vi "GetWindowHandle.vi"(8 "错误输入（无错误）":errorcluster, 11 "Front Panel.Title":string) -> (0 "错误输出":errorcluster, 3 "WindowHandle":u32)   [LabVIEW 2018, in "Win32API.lvlib"]
uses:
  Win32API.lvlib
  user32.dll
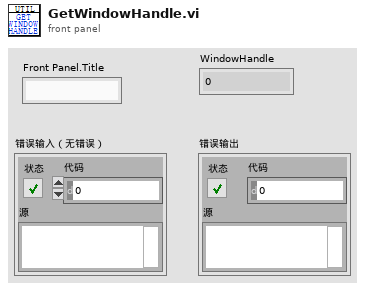
[diagram p1: front panel]
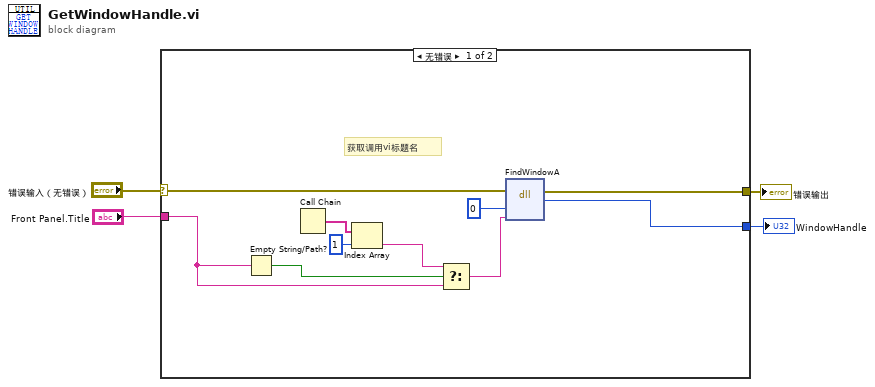
[diagram p0: block diagram]
diagram:
  n1 = case shown="无错误" "错误输入（无错误）" {
    selector: "错误输入（无错误）" -> [w12 w15]
    tunnel: [w14 _] -> w4
    tunnel: "Front Panel.Title" -> [w9 _]
    tunnel: [w13 w15] -> w2
    frame No Error {
      # "获取调用vi标题名"
      n2 = Empty String/Path?(string/path=w9) -> (empty?=w10:bool)
      n3 = Call Chain() -> (call chain=w7:string[])
      n4 = Index Array(array=w7, index=1 ("索引")) -> (element=w5:string)
      n5 = Select(t=w5, s=w10, f=w9) -> (s? t:f=w8:string)
      n6 = dll-call lib="user32.dll" fn="FindWindowA"(error in=w12, "ClassName"=u32 0, "WindowName"=w8) -> (error out=w13:errorcluster, "返回类型"=w14:u32)  [unwired: 4 in, 1 out]
    }
    frame Error {
    }
  }
  "WindowHandle" <- w4
  "错误输出" <- w2
